vi "Inline CRC-16-CCITT.vi"(0 "CRC In":u16 format="%.0x", 1 "CRC-CCITT Type":u16(ring)=65535 items=["CRC-16-CCITT (0x1D0F)"=7439, "CRC-16-CCITT (0xFFFF)"=65535, "CRC-16-CCITT (XModem)"=0], 5 "Reset":bool, 7 "Data":u8 format="%.0x", 11 "error in (no error)":errorcluster) -> (4 "CRC":u16 format="%.0x", 15 "error out":errorcluster)   [LabVIEW 2019]
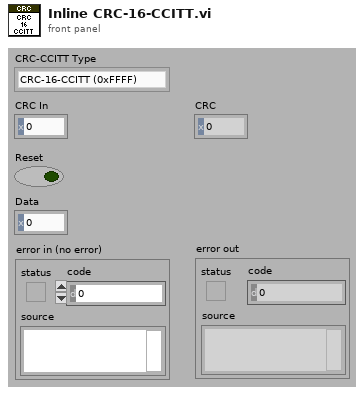
[diagram p1: front panel]
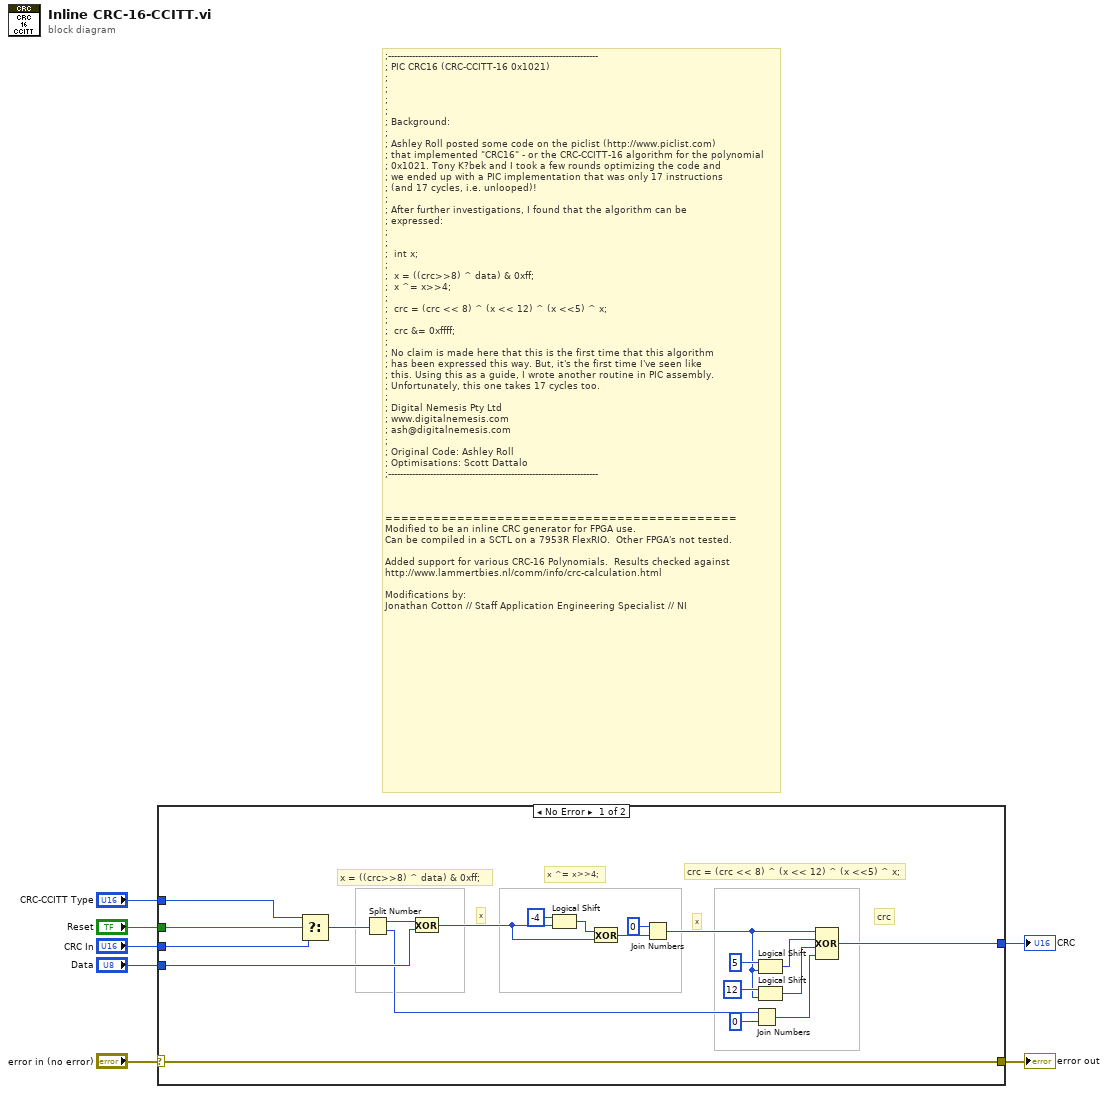
[diagram p0: block diagram]
diagram:
  # ";----------------------------------------------------------------------\n; PIC CRC16 (CRC-CCITT-16 0x1021)\n;\n;\n; \n;\n; Background:\n;\n; Ashley Roll posted some code on the piclist (http://www.piclist.com)\n; that implemented \"CRC16\" - or the CRC-CCITT-16 algorithm for the polynomial\n; 0x1021. Tony K?bek and I took a few rounds optimizing the code and\n; we ended up with a PIC implementation that was only 17 instructions\n; (and 17 cycles, i.e. unlooped)!\n;\n; After further investigations, I found that the algorithm can be \n; expressed:\n;\n;\n;  int x;\n;\n;  x = ((crc>>8) ^ data) & 0xff;\n;  x ^= x>>4;\n;\n;  crc = (crc << 8) ^ (x << 12) ^ (x <<5) ^ x;\n;\n;  crc &= 0xffff;\n;\n; No claim is made here that this is the first time that this algorithm\n; has been expressed this way. But, it's the first time I've seen like\n; this. Using this as a guide, I wrote another routine in PIC assembly.\n; Unfortunately, this one takes 17 cycles too.\n;\n; Digital Nemesis Pty Ltd\n; www.digitalnemesis.com\n; ash@digitalnemesis.com\n;\n; Original Code: Ashley Roll\n; Optimisations: Scott Dattalo\n;----------------------------------------------------------------------\n\n\n\n============================================\nModified to be an inline CRC generator for FPGA use.\nCan be compiled in a SCTL on a 7953R FlexRIO.  Other FPGA's not tested.\n\nAdded support for various CRC-16 Polynomials.  Results checked against\nhttp://www.lammertbies.nl/comm/info/crc-calculation.html\n\nModifications by:\nJonathan Cotton // Staff Application Engineering Specialist // NI"
  n1 = case shown="No Error" "error in (no error)" {
    selector: "error in (no error)" -> [w26 w29]
    tunnel: "Data" -> [w28 _]
    tunnel: "Reset" -> [w27 _]
    tunnel: [w25 _] -> w5
    tunnel: [w26 w29] -> w3
    tunnel: "CRC-CCITT Type" -> [w9 _]
    tunnel: "CRC In" -> [w8 _]
    frame No Error {
      # "crc"
      # "crc = (crc << 8) ^ (x << 12) ^ (x <<5) ^ x;"
      # "x"
      # "x ^= x>>4;"
      # "x"
      # "x = ((crc>>8) ^ data) & 0xff;"
      n2 = Select(t=w9, s=w27, f=w8) -> (s? t:f=w10:u16)
      n3 = Split Number(x=w10) -> (hi(x)=w24:u8, lo(x)=w13:u8)
      n4 = Exclusive Or(1:w28, 2:w24) -> (0:w21:u8)
      n5 = Logical Shift(y=i8 -4, x=w21) -> (x << y=w22:u8)
      n6 = Exclusive Or(1:w21, 2:w22) -> (0:w20:u8)
      n7 = Join Numbers(hi=u8 0, lo=w20) -> ((hi.lo)=w15:u16)
      n8 = Join Numbers(hi=w13, lo=u8 0) -> ((hi.lo)=w11:u16)
      n9 = Logical Shift(y=i8 5, x=w15) -> (x << y=w17:u16)
      n10 = Logical Shift(y=i8 12, x=w15) -> (x << y=w14:u16)
      n11 = Compound Arithmetic op=XOR(w15, w17, w14, w11) -> (w25:u16)
    }
    frame Error {
    }
  }
  "CRC" <- w5
  "error out" <- w3
